vi "数值值时间字符串.vi"(10 "数值":dbl, 11 "String输入":refnum<vi>) -> ()   [LabVIEW 2014]
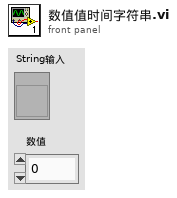
[diagram p1: front panel]
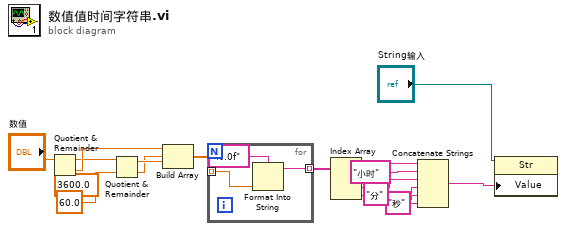
[diagram p0: block diagram]
diagram:
  n1 = Quotient & Remainder(x="数值", y=3600.0) -> (x-y*floor(x/y)=w3:dbl, floor(x/y)=w5:dbl)
  n2 = Quotient & Remainder(x=w3, y=60.0) -> (x-y*floor(x/y)=w7:dbl, floor(x/y)=w6:dbl)
  n3 = Build Array(w5, w6, w7) -> (w8:dbl[])
  n4 = for {
    tunnel: w8 -> [w20] mode=indexing
    tunnel: [w18] -> w9 mode=indexing
    n5 = Format Into String(format string="%.0f" ("格式字符串"), w20) -> (resulting string=w18:string)  [unwired: 2 in, 1 out]
  }
  n6 = Index Array(array=w9) -> (element #1=w10:string, element #2=w12:string, element #3=w14:string)  [unwired: 3 in]
  n7 = Concatenate Strings(w10, "小时" ("字符串"), w12, "分" ("字符串"), w14, "秒" ("字符串")) -> (w16:string)
  n8 = property class="Str"(reference="String输入", "Value"=w16) -> ()  [unwired: 1 in, 2 out]
